vi "Read Action Type and Number.vi"(8 "error in (no error)":errorcluster, 11 "Project Action in":refnum<class "Project Action.lvclass">) -> (0 "error out":errorcluster, 1 "Action Number":i32[](array[numeric]), 2 "Build Step":T1, 3 "Project Action out":refnum<class "Project Action.lvclass">)   [LabVIEW 2019, in "ProjectBuilder.lvlib" / "Project Action.lvclass"]
doc: "Read 'Action Type' and 'Action Number' from the private data."
uses:
  Project Action.lvclass
  Ctl/Ctl_Build Steps.ctl
  ProjectBuilder.lvlib
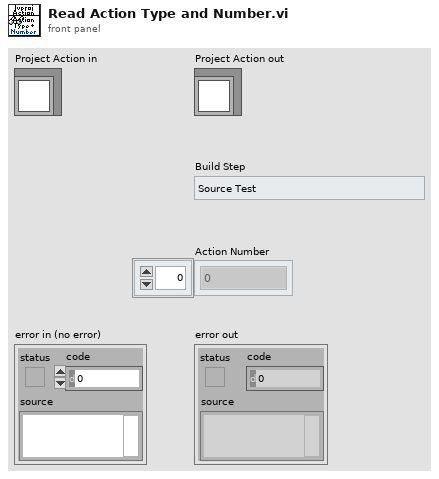
[diagram p1: front panel]
types:
  T1 = typedef "ProjectBuilder.lvlib/Ctl_Build Steps.ctl" = enum16{"Source Test", "Build", "Post-Build Test", "Deploy", "Report"}
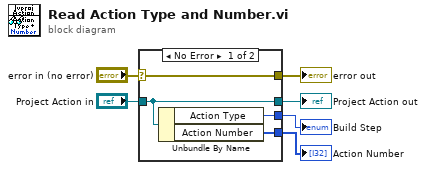
[diagram p0: block diagram]
diagram:
  n1 = case shown="No Error" "error in (no error)" {
    selector: "error in (no error)" -> [w10 w11]
    tunnel: [w10 w11] -> w5
    tunnel: [w9 w12] -> w3
    tunnel: "Project Action in" -> [w9 w12]
    tunnel: [w8 _] -> w2
    tunnel: [w7 _] -> w1
    frame No Error {
      n2 = Unbundle By Name(w9) -> ("Action Type"=w8:T1, "Action Number"=w7:i32[])
    }
    frame Error {
    }
  }
  "error out" <- w5
  "Project Action out" <- w3
  "Build Step" <- w2
  "Action Number" <- w1
